vi "fir_test_reconfig.vi"() -> ()   [LabVIEW 2013]
uses:
  <vilib>/measure/maspectr.llb/Power Spectrum and PSD Export Mode.ctl
  <vilib>/measure/maspectr.llb/FFT Power Spectrum and PSD for 1 Chan.vi
  <vilib>/measure/NI_MABase.lvlib
  <vilib>/measure/NI_MAPro.lvlib
panel:
  out "Array":i32[](array[numeric])
  out "Waveform Graph out":dbl[](graph)
  out "Power spectrum in":cluster{"f0":dbl, "df":dbl, "magnitude":dbl[]}(graph)
  out "Power spectrum":cluster{"f0":dbl, "df":dbl, "magnitude":dbl[]}(graph)
  out "Waveform Graph":dbl[](graph)
  out "# of Iterations":i32
  out "# of samples":i32
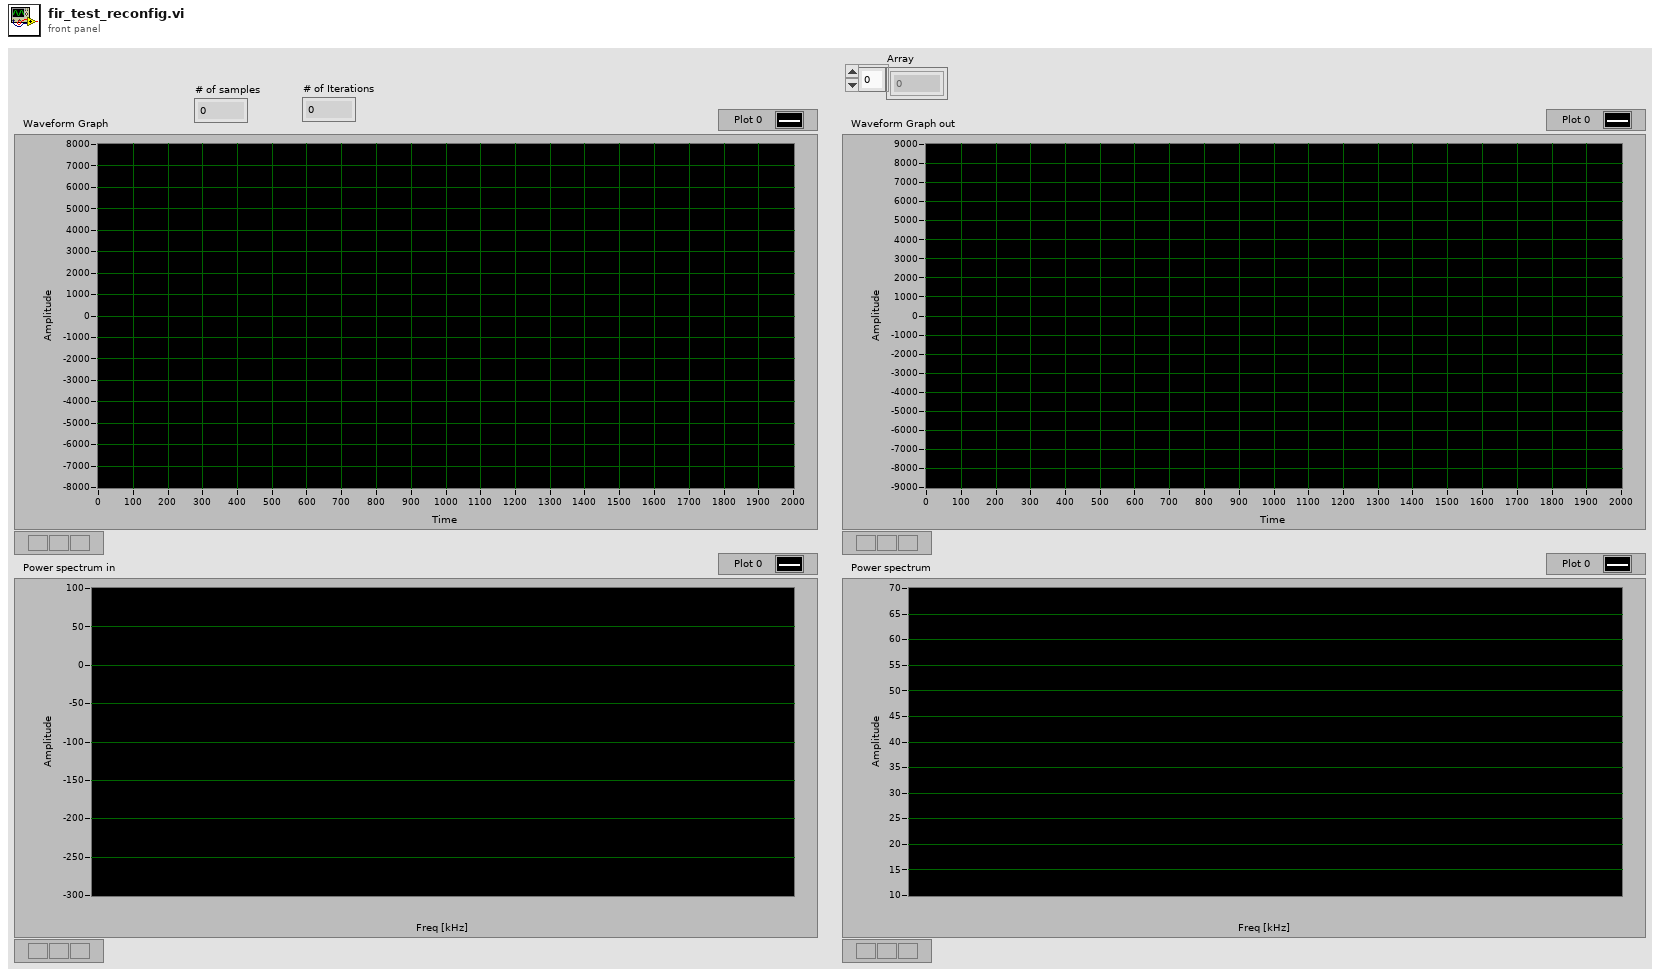
[diagram p1: front panel]
types:
  T1 = typedef "NI_MAPro.lvlib/Power Spectrum and PSD Export Mode.ctl" = u16
  T2 = cluster{"frequency":dbl, "amplitude":dbl, "phase":dbl}[]
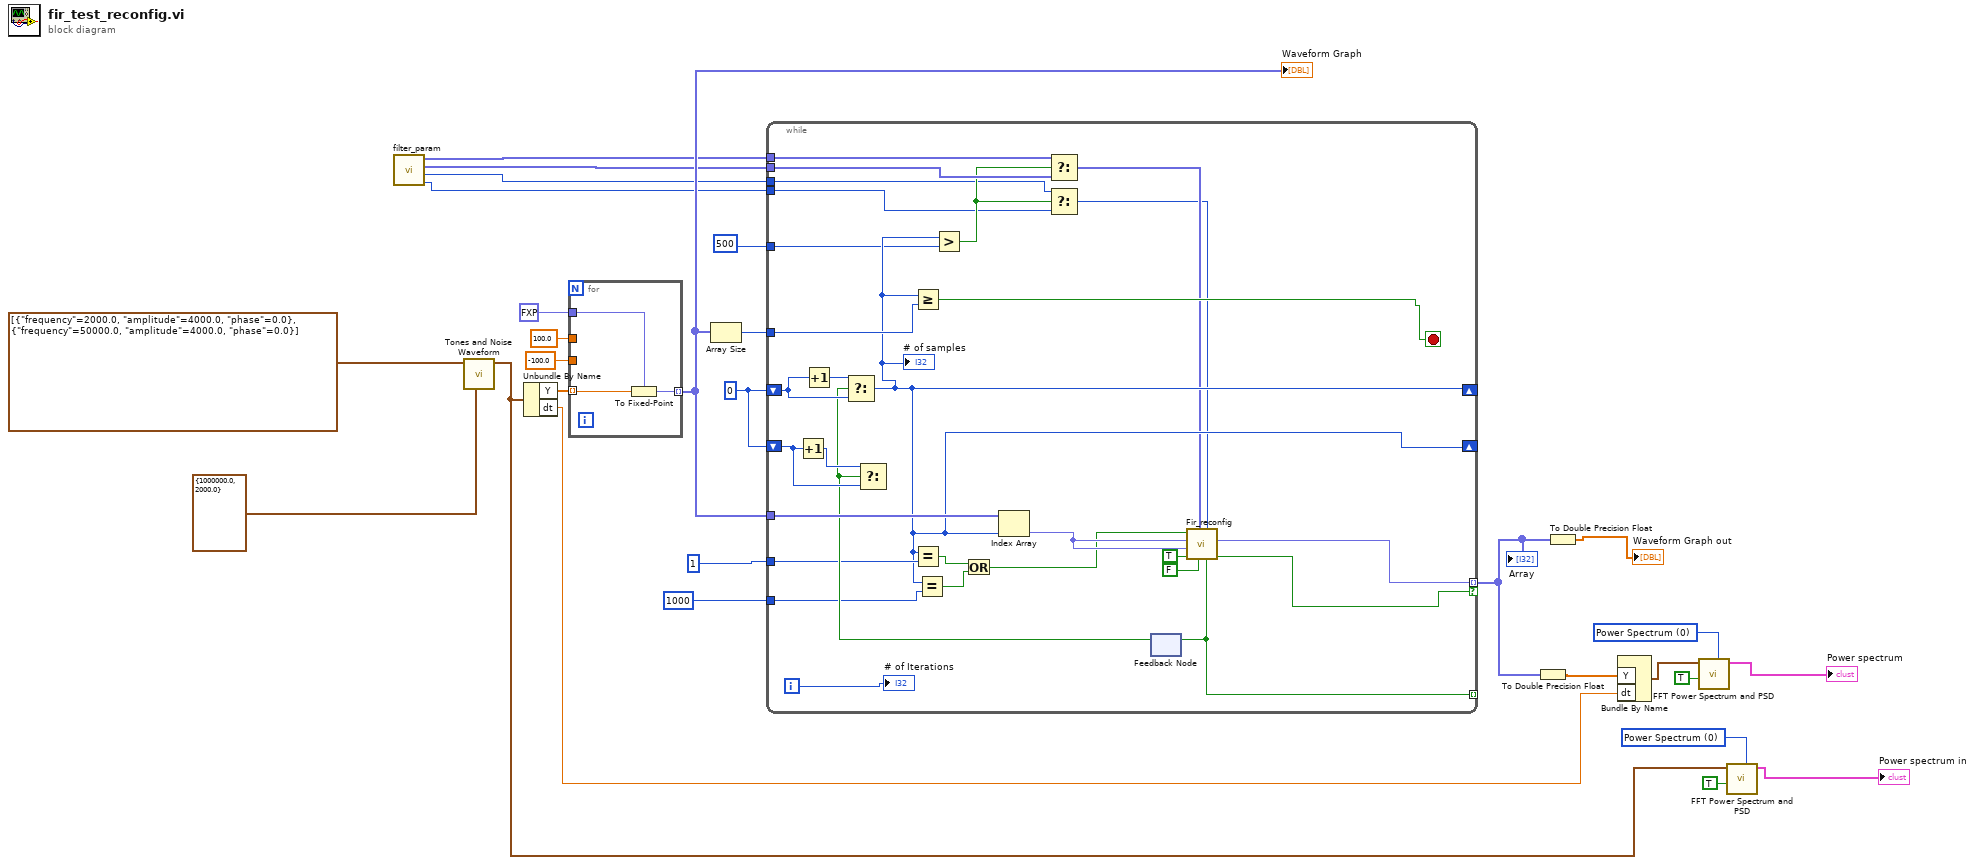
[diagram p0: block diagram]
diagram:
  w16 = T1 0 items=["Power Spectrum", "Power Spectral Density"] ("export mode")
  w22 = T1 0 items=["Power Spectrum", "Power Spectral Density"] ("export mode")
  w24 = 0 ("samples")
  n1 = call "filter_param.vi"() -> ("shift 0.1"=w1:i32, "shift 0.5"=w2:i32, "Coeffs Fs=0.1"=w6:fxp<+/-,18,18>[], "Coeffs Fs=0.5"=w4:fxp<+/-,18,18>[])  [unwired: 8 in]
  n2 = call <vilib>:"Tones and Noise Waveform.vi"("sampling info"=cluster{"Fs":dbl, "#s":dbl} {"Fs"=1000000.0, "#s"=2000.0}, "tones"=T2 [{"frequency"=2000.0, "amplitude"=4000.0, "phase"=0.0}, {"frequency"=50000.0, "amplitude"=4000.0, "phase"=0.0}]) -> ("signal out"=w15:waveform(dbl))  [unwired: 8 in, 1 out]
  n3 = Unbundle By Name(w15) -> ("Y"=w20:dbl[], "dt"=w8:dbl)
  n4 = for {
    tunnel: w20 -> [w29] mode=indexing
    tunnel: fxp<+/-,16,14> 0.0 ("fixed-point type") -> [w31]
    tunnel: [w30] -> w12 mode=indexing
    tunnel: 100.0 -> [_]
    tunnel: -100.0 -> [_]
    n5 = To Fixed-Point(fixed-point type=w31, number=w29) -> (fixed-point=w30:fxp<+/-,16,14>)
  }
  "Waveform Graph" <- w12
  n6 = Array Size(array=w12) -> (size(s)=w25:i32)
  n7 = while {
    tunnel: w12 -> [w60]
    shift-right: [w42] -> _
    shift-left: w24 -> [w58]
    shift-right: [w42] -> _
    shift-left: w24 -> [w56]
    tunnel: [w36] -> w13 mode=indexing if=w49
    tunnel: w25 -> [w54]
    tunnel: 1 ("y") -> [w50]
    tunnel: w6 -> [w40]
    tunnel: [w48] -> _ mode=indexing
    tunnel: 1000 ("y") -> [w45]
    tunnel: w4 -> [w43]
    tunnel: 500 ("y") -> [w41]
    tunnel: w2 -> [w34]
    tunnel: w1 -> [w33]
    i -> [w47]
    stop <- w55 stop-if-true
    n8 = Increment(x=w58) -> (x+1=w59:i32)
    n9 = Increment(x=w56) -> (x+1=w57:i32)
    n10 = feedback #1() -> (w51:bool)  [unwired: 1 in]
    n11 = Select(t=w57, s=w51, f=w56) -> (s? t:f=w42:i32)
    "# of samples" <- w42
    n12 = Select(t=w59, s=w51, f=w58) -> ()  [unwired: 1 out]
    n13 = Greater Or Equal?(x=w42, y=w54) -> (x >= y?=w55:bool)
    n14 = Equal?(x=w42, y=w50) -> (x = y?=w39:bool)
    n15 = Equal?(x=w42, y=w45) -> (x = y?=w44:bool)
    n16 = Greater?(x=w42, y=w41) -> (0:w35:bool)
    n17 = Or(x=w39, y=w44) -> (x .or. y?=w38:bool)
    n18 = Index Array(array=w60, index=w42) -> (element=w53:fxp<+/-,16,14>)
    n19 = Select(t=w43, s=w35, f=w40) -> (s? t:f=w37:fxp<+/-,18,18>[])
    n20 = Select(t=w34, s=w35, f=w33) -> (s? t:f=w32:i32)
    n21 = call "Fir_reconfig.vi"("new shift"=w32, "reset"=FALSE, 7:"new coeffs"=w37, "valid in"=TRUE, "Q in"=w53, "I in"=w53, 11:"new coeffs"=w38) -> ("valid out"=w49:bool, "I out"=w36:fxp<+/-,16,14>, "ready for input"=w48:bool)  [unwired: 1 in, 1 out]
    n22 = feedback-in #1(w48) -> ()
    "# of Iterations" <- w47
  }
  "Array" <- w13
  n23 = To Double Precision Float(number=w13) -> (double precision float=w18:dbl[])
  n24 = To Double Precision Float(number=w13) -> (double precision float=→"Waveform Graph out":dbl[])
  n25 = Bundle By Name("Y"=w18, "dt"=w8) -> (w23:waveform(dbl))  [unwired: 1 in]
  n26 = call-poly <vilib>:"FFT Power Spectrum and PSD.vi"("export mode"=w22, "dB On (F)"=TRUE, "time signal"=w23) -> ("Power Spectrum / PSD"=→"Power spectrum":cluster{"f0":dbl, "df":dbl, "magnitude":dbl[]})  [unwired: 5 in, 3 out]
  n27 = call-poly <vilib>:"FFT Power Spectrum and PSD.vi"("export mode"=w16, "dB On (F)"=TRUE, "time signal"=w15) -> ("Power Spectrum / PSD"=→"Power spectrum in":cluster{"f0":dbl, "df":dbl, "magnitude":dbl[]})  [unwired: 5 in, 3 out]
